vi "tempMeasurement1.vi"() -> ()   [LabVIEW 2011]
panel:
  in  "output cluster":cluster{dbl[], dbl[]}(graph)
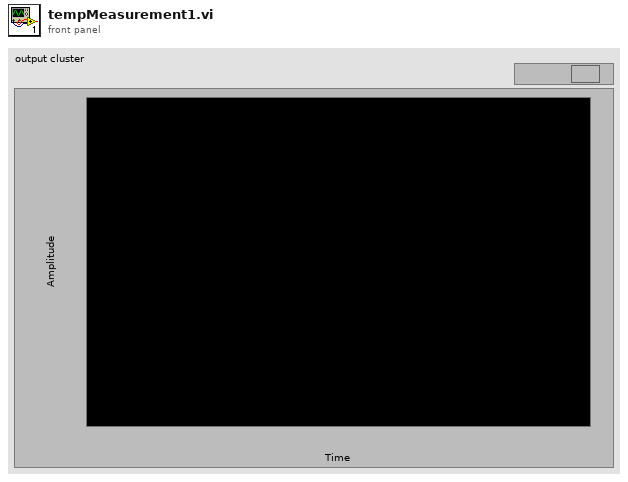
[diagram p1: front panel]
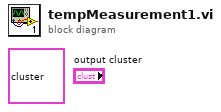
[diagram p0: block diagram]
diagram:
  (unwired) cluster{dbl[], dbl[]} {array[1084 elements], array[1084 elements]} ("output cluster")
